vi "NewPosIndex.vi"(8 "Array 4":u16[][](array[numeric]), 9 "Snake Positions":cluster{"R":i32, "C":i32}[](array[cluster]), 10 "c":i32, 11 "r":i32) -> (2 "newc":i32, 3 "newr":i32)   [LabVIEW 2014]
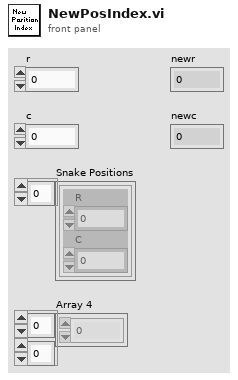
[diagram p1: front panel]
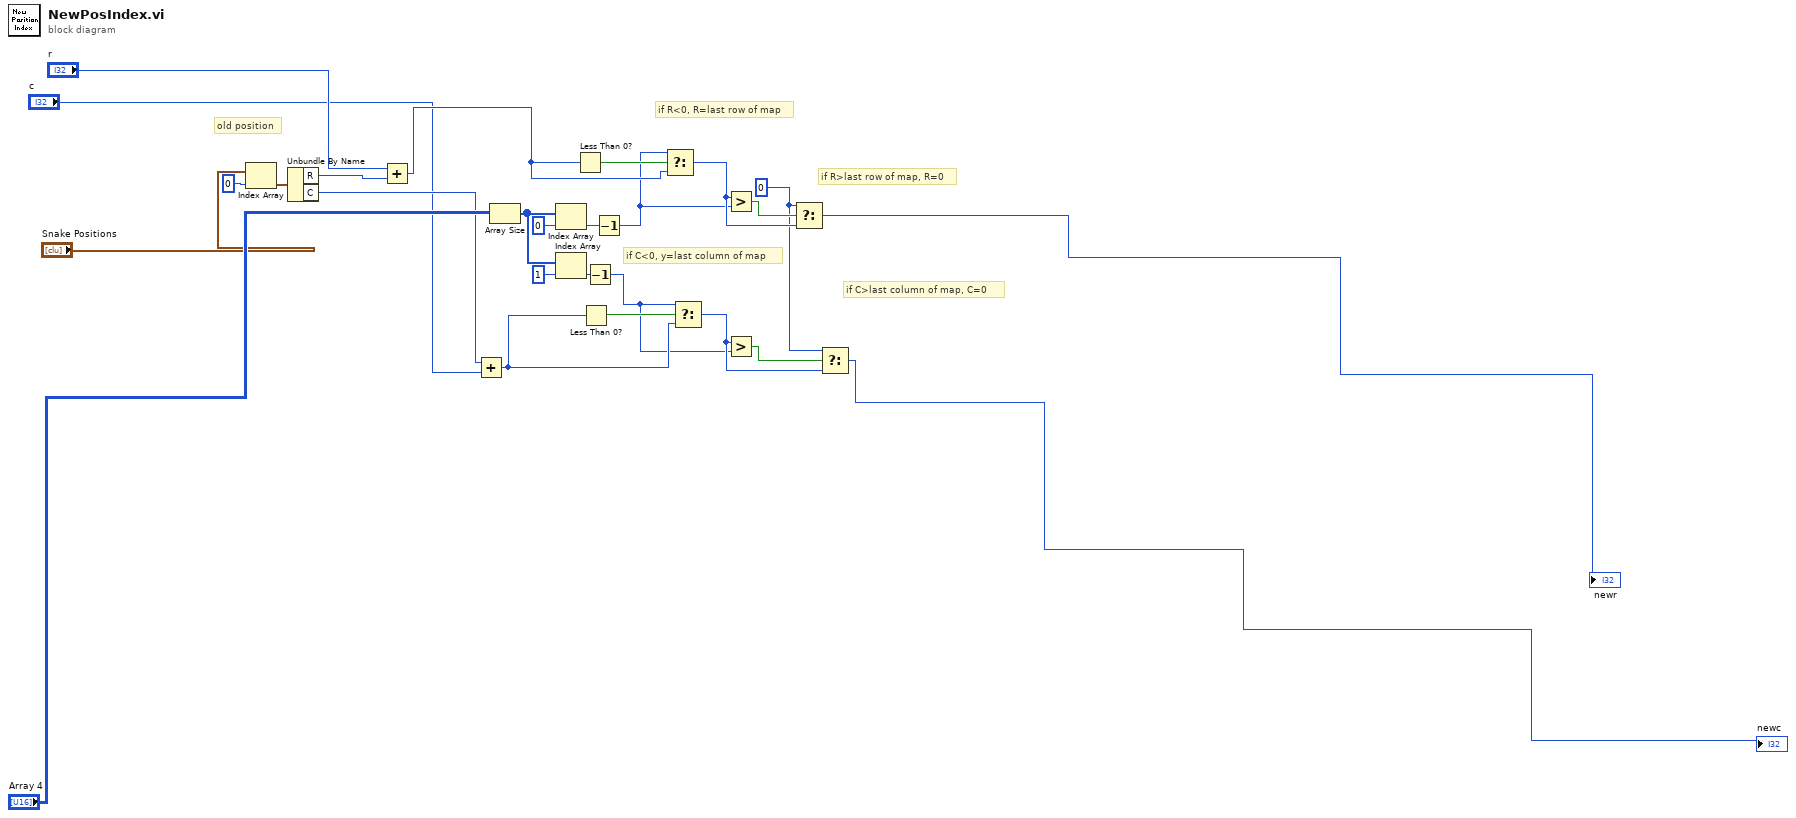
[diagram p0: block diagram]
diagram:
  w11 = 0 ("index")
  # "if C>last column of map, C=0"
  # "if C<0, y=last column of map"
  # "if R>last row of map, R=0"
  # "if R<0, R=last row of map"
  # "old position"
  n1 = Index Array(array="Snake Positions", index=0) -> (element=w6:cluster{"R":i32, "C":i32})
  n2 = Unbundle By Name(w6) -> ("R"=w4:i32, "C"=w2:i32)
  n3 = Add(x="r", y=w4) -> (x+y=w22:i32)
  n4 = Add(x=w2, y="c") -> (x+y=w23:i32)
  n5 = Array Size(array="Array 4") -> (size(s)=w19:i32[])
  n6 = Index Array(array=w19, index=0) -> (element=w17:i32)
  n7 = Index Array(array=w19, index=1) -> (element=w13:i32)
  n8 = Less Than 0?(x=w22) -> (x < 0?=w21:bool)
  n9 = Less Than 0?(x=w23) -> (x < 0?=w14:bool)
  n10 = Decrement(x=w13) -> (x-1=w8:i32)
  n11 = Decrement(x=w17) -> (x-1=w9:i32)
  n12 = Select(t=w9, s=w21, f=w22) -> (s? t:f=w15:i32)
  n13 = Select(t=w8, s=w14, f=w23) -> (s? t:f=w10:i32)
  n14 = Greater?(x=w15, y=w9) -> (0:w16:bool)
  n15 = Greater?(x=w10, y=w8) -> (0:w12:bool)
  n16 = Select(t=w11, s=w16, f=w15) -> (s? t:f=→"newr":i32)
  n17 = Select(t=w11, s=w12, f=w10) -> (s? t:f=→"newc":i32)
